vi "Lockin_Metrics.vi"() -> ()   [LabVIEW 2019]
uses:
  src/Instrument.Lockin/Typedefs/Results Type--Enum.ctl
  src/Instrument.Lockin/Instrument.Lockin.lvclass
  src/Instrument.DAQ/Typedefs/DAQ.Sampling.Sampling--Cluster.ctl
  src/Instrument.DAQ/Instrument.DAQ.lvclass
panel:
  out "#s":i32
  in  "Fs":dbl[](array[numeric])=[204800.0, 180000.0, 160000.0, 140000.0, 120000.0, 102400.0, 90000.0, 80000.0, 70000.0, 60000.0, 51200.0, 40000.0, 30000.0, 25600.0, 20000.0, 15000.0, 12800.0]
  out "N":i32=97280
  out "XY Graph 4":cluster{dbl[], dbl[]}(graph)={[6.309573444801933, 7.943282347242816, 10.0, 12.589254117941675, 15.848931924611142, 19.952623149688797, 25.11886431509581, 31.622776601683793, 39.810717055349734, 50.11872336272725, 63.09573444801933, 79.43282347242817, 100.0], [204800.0, 204800.0, 204800.0, 204800.0, 204800.0, 204800.0, 204800.0, 204800.0, 204800.0, 204800.0, 204800.0, 204800.0, 204800.0, 204800.0, 204800.0, 204800.0, 204800.0, 204800.0, 204800.0, 204800.0, 204800.0, 204800.0, 204800.0, 204800.0, 204800.0, 204800.0, 204800.0, 204800.0, 102400.0, 102400.0, 102400.0, 102400.0, 102400.0, 102400.0, 102400.0, 102400.0, 102400.0, 102400.0, 102400.0, 102400.0, 102400.0]}
  out "XY Graph 3":cluster{dbl[], i32[]}(graph)={[6.309573444801933, 7.943282347242816, 10.0, 12.589254117941675, 15.848931924611142, 19.952623149688797, 25.11886431509581, 31.622776601683793, 39.810717055349734, 50.11872336272725, 63.09573444801933, 79.43282347242817, 100.0], [20480, 20480, 20480, 20480, 20480, 20480, 20480, 20480, 20480, 20480, 20480, 20480, 20480, 20480, 20480, 20480, 20480, 20480, 20480, 20480, 20480, 20480, 20480, 20480, 20480, 20480, 20480, 20480, 20480, 20480, 20480, 20480, 20480, 20480, 20480, 20480, 20480, 20480, 20480, 20480, 20480]}
  in  "N start":dbl=102400.0
  in  "N end":dbl=20480.0
  in  "N step":dbl=5120.0
  out "XY Graph 2":cluster{i32[], dbl[]}(graph)={[20480, 20480, 20480, 20480, 20480, 20480, 20480, 20480, 20480, 20480, 20480, 20480, 20480, 20480, 20480, 20480, 20480, 20480, 20480, 20480, 20480, 20480, 20480, 20480, 20480, 20480, 20480, 20480, 20480, 20480, 20480, 20480, 20480, 20480, 20480, 20480, 20480, 20480, 20480, 20480], [1729.70703125, 1761.4453125, 1746.765625, 1742.35546875, 1749.078125, 1754.49609375, 1755.8125, 1764.29296875, 1766.453125, 1771.67578125, 1791.0546875, 1829.34375]}
  in  "stop":bool
  out "Frequency (Hz)":dbl=100.0
  out "XY Graph":cluster{dbl[], dbl[]}[](graph)=[{[6.309573444801933, 7.943282347242816, 10.0, 12.589254117941675, 15.848931924611142, 19.952623149688797, 25.11886431509581, 31.622776601683793, 39.810717055349734, 50.11872336272725, 63.09573444801933, 79.43282347242817, 100.0], [-0.0559482465843852, -0.114647989593913, -0.08823088751996, -0.117279915043384, -0.1395285316251, -0.190130151485401, -0.229514920362016, -0.287924590215895, -0.362077203901885, -0.460392693393047, -0.572833357365753, 0.0, 0.0]}]
  in  "f step":dbl=0.1
  in  "f end":dbl=3.5
  in  "f start":dbl=3.3
  # "Sweep frequency:"
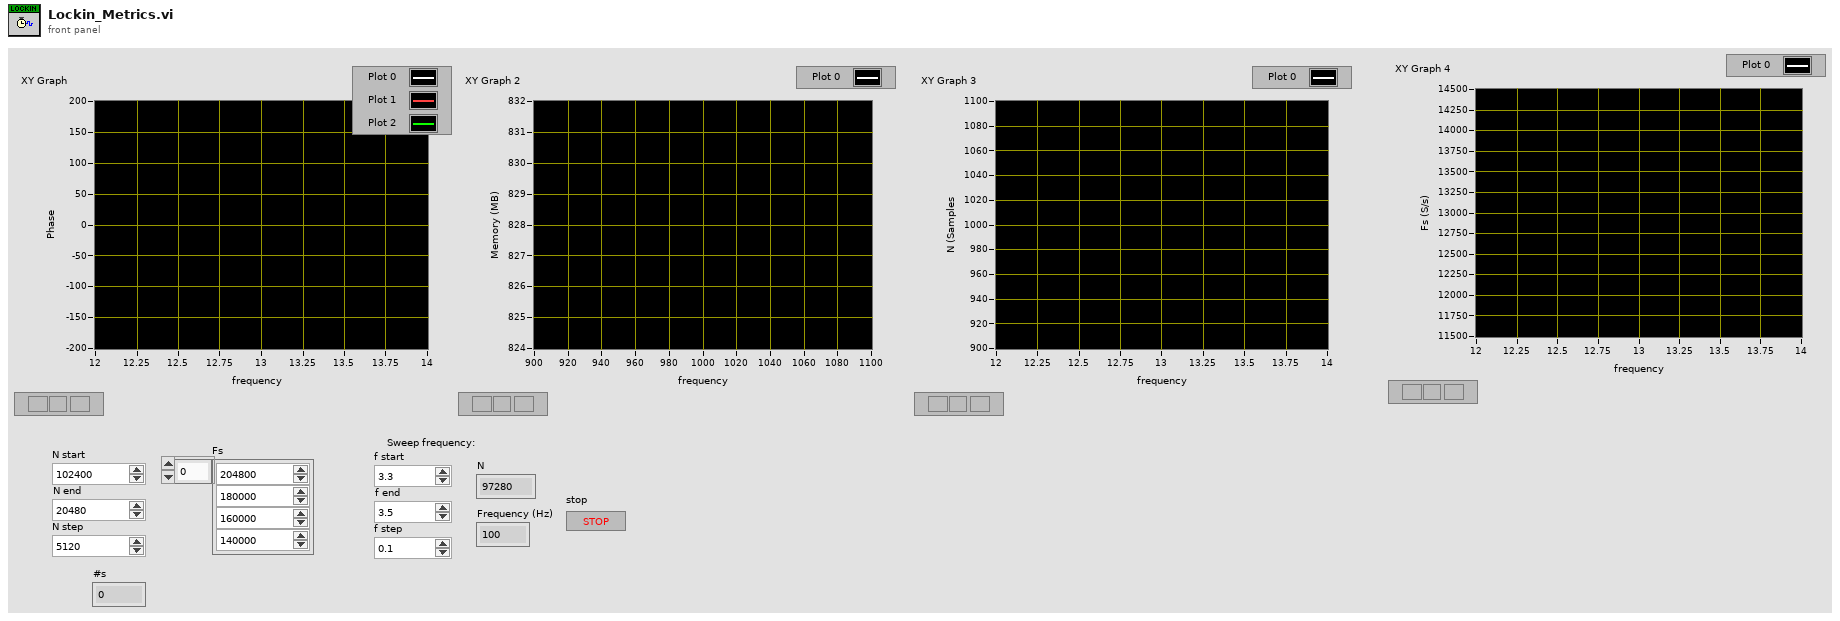
[diagram p1: front panel]
types:
  T1 = typedef "Instrument.Lockin.lvlib/Instrument.DAQ.lvclass/DAQ.Sampling.Sampling--Cluster.ctl" = cluster{"Fs":dbl, "#s":i32}
  T2 = typedef "Instrument.Lockin.lvlib/Instrument.Lockin.lvclass/Results Type--Enum.ctl" = enum16{"X", "Y", "R", "Theta", "Mean"}
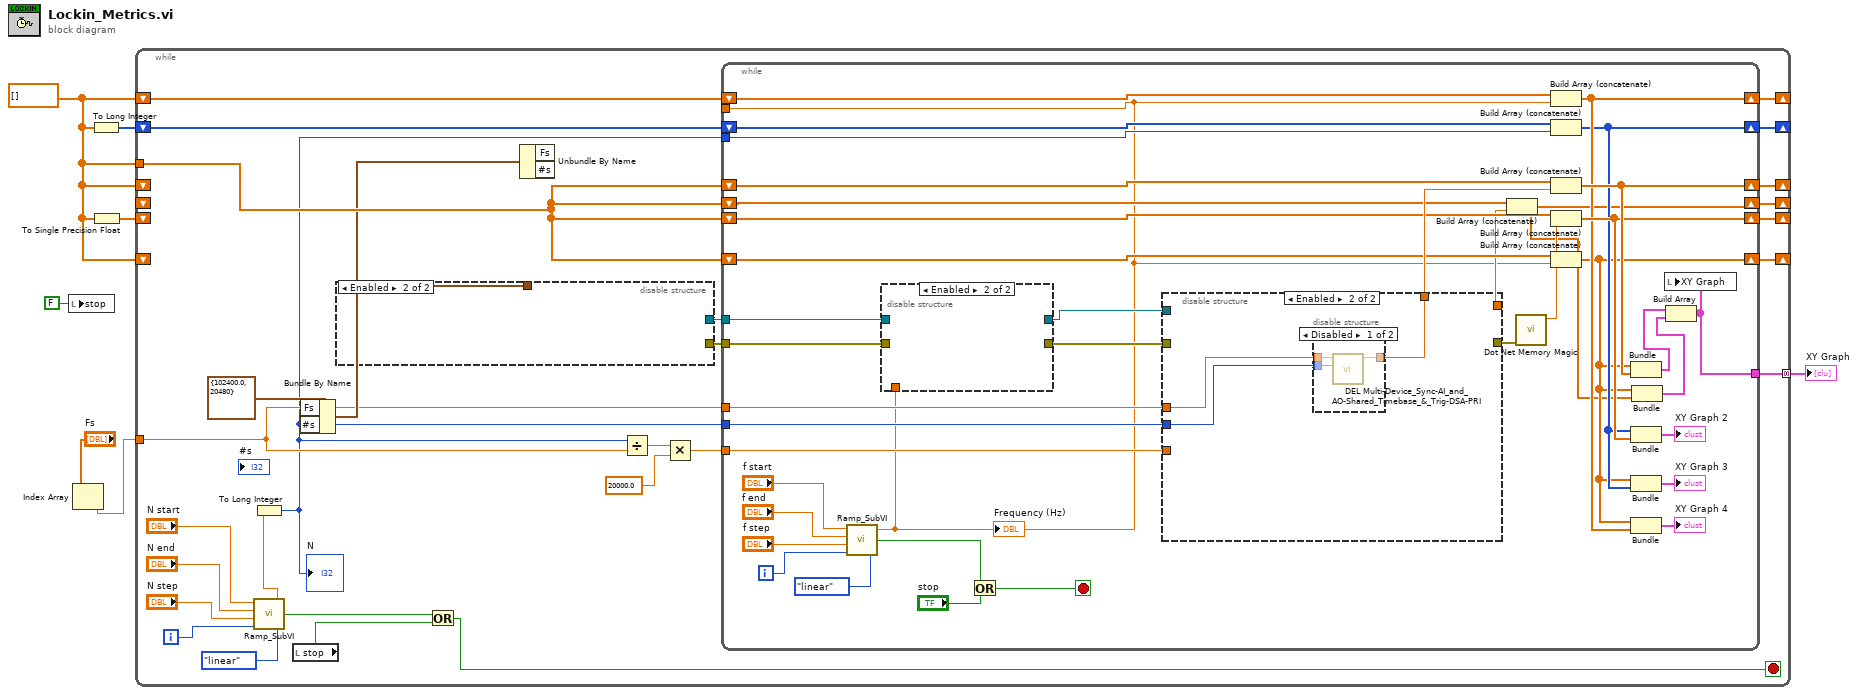
[diagram p0: block diagram]
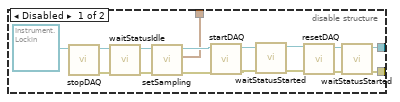
[diagram p2: hidden frame]
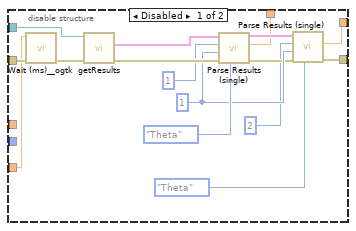
[diagram p3: hidden frame]
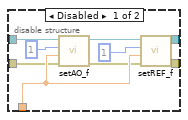
[diagram p5: hidden frame]
diagram:
  w3 = dbl[] []
  n1 = local write "stop"(FALSE ("stop")) -> ()
  n2 = Index Array(array="Fs") -> (element=w2:dbl)  [unwired: 1 in]
  n3 = To Long Integer(number=w3) -> (32bit integer=w7:i32[])
  n4 = To Single Precision Float(number=w3) -> (single precision float=w5:sgl[])
  n5 = while {
    shift-right: [w25] -> _
    shift-left: w3 -> [w19]
    shift-right: [w22] -> _
    shift-left: w7 -> [w20]
    shift-right: [w21] -> _
    shift-left: w3 -> [_]
    shift-right: [w23] -> _
    shift-left: w3 -> [_]
    shift-right: [w24] -> _
    shift-left: w5 -> [_]
    tunnel: [w18] -> w4 mode=concatenating
    tunnel: w3 -> [w15]
    tunnel: w2 -> [w10]
    shift-right: [w16] -> _
    shift-left: _ -> [_]
    i -> [w31]
    stop <- w17 stop-if-true
    n6 = call <userlib>:"Ramp_SubVI.vi"("Enum"=enum16{"linear", "power"}."linear", "index"=w31, "step"="N step", "end"="N end", "start"="N start") -> ("Stop?"=w30:bool, "Numeric"=w9:dbl)
    n7 = To Long Integer(number=w9) -> (32bit integer=w8:i32)
    "N" <- w8
    n8 = local read "stop"() -> (w29:bool)
    n9 = Bundle By Name(cluster=T1 {"Fs"=102400.0, "#s"=20480} ("Sampling"), "Fs"=w10, "#s"=w8) -> (w11:T1)
    n10 = disable-structure shown="Enabled" {
      disable-tunnel: [w45 _] -> w27
      disable-tunnel: [w44 _] -> w26
      disable-tunnel: w11 -> [w36 _]
      frame Disabled {
        n11 = call-dynamic "stopDAQ.vi"("Instrument.Lockin in"=refnum<class "Instrument.Lockin.lvclass"> refnum) -> ("error out"=w50:errorcluster, "Instrument.Lockin out"=w51:refnum<class "Instrument.Lockin.lvclass">)  [unwired: 9 in]
        n12 = call-dynamic "waitStatusIdle.vi"("error in (no error)"=w50, "Instrument.Lockin in"=w51) -> ("error out"=w49:errorcluster, "Instrument.Lockin out"=w48:refnum<class "Instrument.Lockin.lvclass">)  [unwired: 8 in]
        n13 = call-dynamic "setSampling.vi"("error in (no error)"=w49, "sampling"=w36, "Instrument.Lockin in"=w48) -> ("error out"=w47:errorcluster, "Instrument.Lockin out"=w46:refnum<class "Instrument.Lockin.lvclass">)  [unwired: 7 in]
        n14 = call-dynamic "startDAQ.vi"("error in (no error)"=w47, "Instrument.Lockin in"=w46) -> ("error out"=w39:errorcluster, "Instrument.Lockin out"=w41:refnum<class "Instrument.Lockin.lvclass">)  [unwired: 8 in]
        n15 = call-dynamic "waitStatusStarted.vi"("error in (no error)"=w39, "Instrument.Lockin in"=w41) -> ("error out"=w38:errorcluster, "Instrument.Lockin out"=w40:refnum<class "Instrument.Lockin.lvclass">)  [unwired: 8 in]
        n16 = call-dynamic "resetDAQ.vi"("error in (no error)"=w38, "Instrument.Lockin in"=w40) -> ("error out"=w42:errorcluster, "Instrument.Lockin out"=w43:refnum<class "Instrument.Lockin.lvclass">)  [unwired: 8 in]
        n17 = call-dynamic "waitStatusStarted.vi"("error in (no error)"=w42, "Instrument.Lockin in"=w43) -> ("error out"=w45:errorcluster, "Instrument.Lockin out"=w44:refnum<class "Instrument.Lockin.lvclass">)  [unwired: 8 in]
      }
      frame Enabled {
      }
    }
    n18 = Or(x=w30, y=w29) -> (x .or. y?=w17:bool)
    n19 = Unbundle By Name(w11) -> ()  [unwired: 2 out]
    n20 = Divide(x=w8, y=w10) -> (x/y=w14:dbl)
    n21 = Multiply(x=w14, y=20000.0) -> (x*y=w12:dbl)
    n22 = while {
      shift-right: [w61] -> w21
      shift-left: w15 -> [w81]
      shift-right: [w77] -> w23
      shift-left: w15 -> [w82]
      shift-right: [w76] -> w24
      shift-left: w15 -> [w78]
      shift-right: [w71] -> w25
      shift-left: w19 -> [w72]
      shift-right: [w66] -> w22
      shift-left: w20 -> [w73]
      tunnel: w27 -> [w67]
      tunnel: w26 -> [w68]
      tunnel: w8 -> [w74]
      tunnel: [w52] -> _
      tunnel: [w56] -> w18
      shift-right: [w58] -> w16
      shift-left: w15 -> [w60]
      tunnel: w12 -> [w55]
      tunnel: w10 -> [w54]
      tunnel: w8 -> [w53]
      i -> [w90]
      stop <- w65 stop-if-true
      n23 = call <userlib>:"Ramp_SubVI.vi"("Enum"=enum16{"linear", "power"}."linear", "index"=w90, "step"="f step", "end"="f end", "start"="f start") -> ("Stop?"=w84:bool, "Numeric"=w52:dbl)
      "Frequency (Hz)" <- w52
      n24 = disable-structure shown="Enabled" {
        disable-tunnel: w52 -> [w120 _]
        disable-tunnel: w68 -> [w119 _]
        disable-tunnel: w67 -> [w118 _]
        disable-tunnel: [w115 _] -> w63
        disable-tunnel: [w114 _] -> w62
        frame Disabled {
          n25 = call-dynamic "setAO_f.vi"("error in (no error)"=w118, "Frequency (Hz)"=w120, "AO Channel"=1, "Instrument.Lockin in"=w119) -> ("error out"=w117:errorcluster, "Instrument.Lockin out"=w116:refnum<class "Instrument.Lockin.lvclass">)  [unwired: 6 in]
          n26 = call-dynamic "setREF_f.vi"("error in (no error)"=w117, "Frequency (Hz)"=w120, "REF Channel"=1, "Instrument.Lockin in"=w116) -> ("error out"=w114:errorcluster, "Instrument.Lockin out"=w115:refnum<class "Instrument.Lockin.lvclass">)  [unwired: 6 in]
        }
        frame Enabled {
        }
      }
      n27 = Or(x=w84, y="stop") -> (x .or. y?=w65:bool)
      n28 = disable-structure shown="Enabled" {
        disable-tunnel: [w97 w107] -> w83
        disable-tunnel: [w96 _] -> w80
        disable-tunnel: w63 -> [w95 _]
        disable-tunnel: w62 -> [w94 _]
        disable-tunnel: [w92 _] -> w59
        disable-tunnel: w55 -> [w91 _]
        disable-tunnel: w54 -> [_ w109]
        disable-tunnel: w53 -> [_ w108]
        frame Disabled {
          w102 = 1 ("Reference Channel")
          n29 = call <userlib>:"Wait (ms)__ogtk.vi"("error in (no error)"=w94, "milliseconds to wait"=w91) -> ("error out"=w106:errorcluster)  [unwired: 8 in, 1 out]
          n30 = call-dynamic "getResults.vi"("error in (no error)"=w106, "Instrument.Lockin in"=w95) -> ("error out"=w104:errorcluster, "Results (Dictionary)"=w105:cluster{"key":string, "value":dbl}[])  [unwired: 6 in, 2 out]
          n31 = call "Parse Results (single).vi"("Type"=Results_Type--Enum."Theta", "error in (no error)"=w104, "Reference Channel"=w102, "AI Channel"=1, "Results (Dictionary)"=w105) -> ("error out"=w99:errorcluster, "Data"=w97:dbl, "Results (Dictionary)"=w100:cluster{"key":string, "value":dbl}[])  [unwired: 3 in, 1 out]
          n32 = call "Parse Results (single).vi"("Type"=Results_Type--Enum."Theta", "error in (no error)"=w99, "Reference Channel"=w102, "AI Channel"=2, "Results (Dictionary)"=w100) -> ("error out"=w96:errorcluster, "Data"=w92:dbl)  [unwired: 3 in, 2 out]
        }
        frame Enabled {
          n33 = disable-structure shown="Disabled" {
            disable-tunnel: w109 -> [w112 _]
            disable-tunnel: w108 -> [w111 _]
            disable-tunnel: [w110 _] -> w107
            frame Disabled {
              n34 = call "DEL Multi-Device_Sync-AI_and_AO-Shared_Timebase_&_Trig-DSA-PRI.vi"("Samples per Channel"=w111, "SampClk.Rate"=w112) -> ("AO - AI"=w110:dbl)  [unwired: 9 in]
            }
            frame Enabled {
            }
          }
        }
      }
      n35 = Build Array (concatenate)(w60, w59) -> (w58:dbl[])
      n36 = call "Dot Net Memory Magic.vi"("error in (no error)"=w80) -> ("Private Memory (MB)"=w79:sgl)  [unwired: 9 in, 1 out]
      n37 = Build Array (concatenate)(w72, w52) -> (w71:dbl[])
      n38 = Build Array (concatenate)(w73, w74) -> (w66:i32[])
      n39 = Build Array (concatenate)(w82, w83) -> (w77:dbl[])
      n40 = Build Array (concatenate)(w78, w79) -> (w76:dbl[])
      n41 = Build Array (concatenate)(w81, w52) -> (w61:dbl[])
      n42 = Bundle(w61, w77) -> (w64:cluster{dbl[], dbl[]})  [unwired: 1 in]
      n43 = Bundle(w66, w76) -> (→"XY Graph 2":cluster{i32[], dbl[]})  [unwired: 1 in]
      n44 = Bundle(w61, w66) -> (→"XY Graph 3":cluster{dbl[], i32[]})  [unwired: 1 in]
      n45 = Bundle(w61, w71) -> (→"XY Graph 4":cluster{dbl[], dbl[]})  [unwired: 1 in]
      n46 = Bundle(w61, w58) -> (w57:cluster{dbl[], dbl[]})  [unwired: 1 in]
      n47 = Build Array(w64, w57) -> (w56:cluster{dbl[], dbl[]}[])
      n48 = local write "XY Graph"(w56) -> ()
    }
  }
  "XY Graph" <- w4
